vi "GetConfigChain.vi"(8 "error in (no error)":errorcluster, 11 "reference in":refnum<class "Switch_Keysight_34934A.lvclass">) -> (0 "error out":errorcluster, 2 "Config out":string[](array[string]), 3 "reference out":refnum<class "Switch_Keysight_34934A.lvclass">)   [LabVIEW 2022 SP3, in "Switch_Keysight_34934A.lvlib" / "Switch_Keysight_34934A.lvclass"]
uses:
  Switch_Keysight_34934A.lvclass
  Components/SwitchBase.lvlibp/SwitchBase.lvclass
  Components/ViPER.lvlibp/ViPER.lvclass
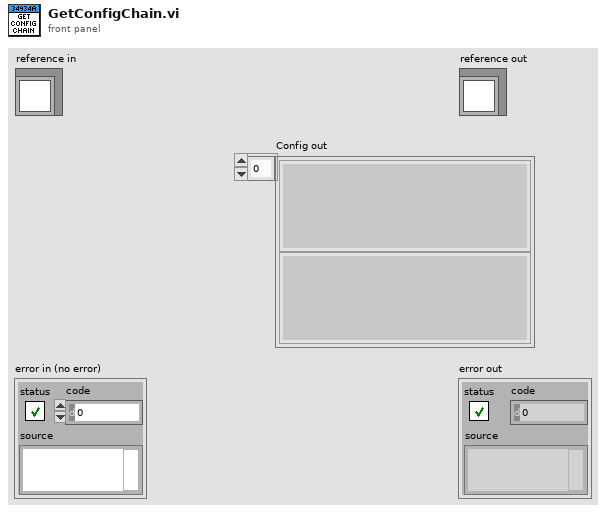
[diagram p1: front panel]
types:
  T1 = typedef "Switch_Keysight_34934A.lvlib/Switch_Keysight_34934A.lvclass/ObjectAttributes.ctl" = cluster{"Config":T2, "VISA ref":refnum<visa-resource-name>, "M1H":bool[][], "M2H":bool[][], "M1L":bool[][], "M2L":bool[][], "route":string, "State":bool[], "StateModBit":bool[], "UpdateEvent":refnum<user-event>}
  T2 = typedef "Switch_Keysight_34934A.lvlib/Switch_Keysight_34934A.lvclass/Config.ctl" = cluster{"VISA":refnum<visa-resource-name>, "Slot":i32, "SwitchMap":cluster{"Name":string, "Route":string[], "UnRoute":string[], "Description":string, "Group":string, "IsGroup":bool}[], "Sim":bool}
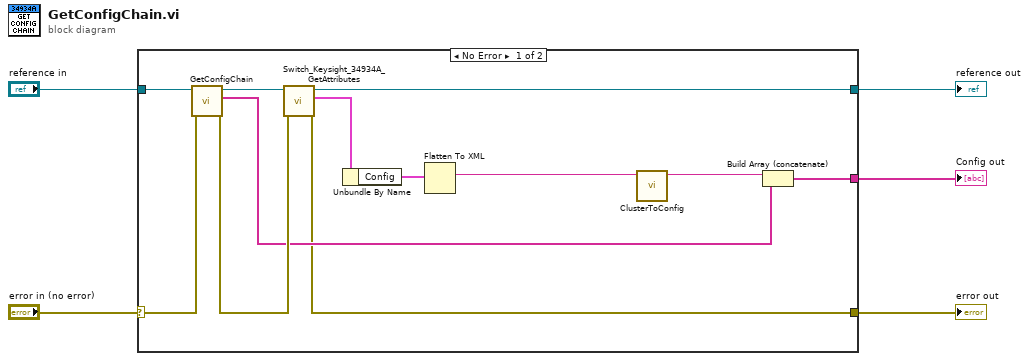
[diagram p0: block diagram]
diagram:
  n1 = case shown="No Error" "error in (no error)" {
    selector: "error in (no error)" -> [w13 w19]
    tunnel: [w6 w19] -> w4
    tunnel: [w11 w18] -> w2
    tunnel: "reference in" -> [w15 w18]
    tunnel: [w8 _] -> w1
    frame No Error {
      n2 = call-parent "GetConfigChain.vi"("error in (no error)"=w13, "reference in"=w15) -> ("error out"=w12:errorcluster, "Config out"=w9:string[], "reference out"=w14:refnum<class "Switch_Keysight_34934A.lvclass">)  [unwired: 7 in]
      n3 = call "Switch_Keysight_34934A_GetAttributes.vi"("error in (no error)"=w12, "reference in"=w14) -> ("error out"=w6:errorcluster, "Data"=w17:T1, "reference out"=w11:refnum<class "Switch_Keysight_34934A.lvclass">)  [unwired: 6 in, 1 out]
      n4 = Unbundle By Name(w17) -> ("Config"=w16:T2)
      n5 = Flatten To XML(6:w16) -> (2:w7:string)
      n6 = call "ClusterToConfig.vi"("Cluster XML"=w7) -> ("Config XML"=w10:string)  [unwired: 10 in]
      n7 = Build Array (concatenate)(w10, w9) -> (w8:string[])
    }
    frame Error {
    }
  }
  "error out" <- w4
  "reference out" <- w2
  "Config out" <- w1
